vi "get trigger out before integration.vi"(8 "error in (no error)":errorcluster, 11 "LineCCD in":refnum<class "LineCCD.lvclass">) -> (0 "error out":errorcluster, 3 "LineCCD out":refnum<class "LineCCD.lvclass">)   [LabVIEW 2012, in "LineCCD.lvclass"]
uses:
  LineCCD.lvclass
  LineCCD.lvclass/LineCCD.ctl
  <instrlib>/ALPHALAS CCD S Series/ALPHALAS CCD S Series.lvlib
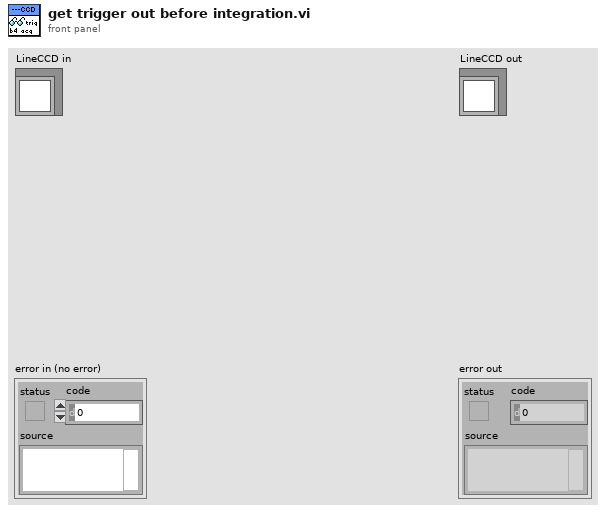
[diagram p1: front panel]
types:
  T1 = typedef "ALPHALAS CCD S Series.lvlib/Trig Out Before Integration.ctl" = u32
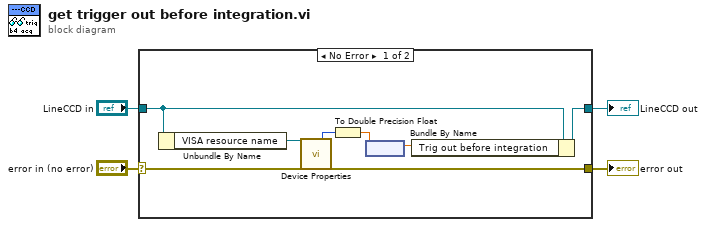
[diagram p0: block diagram]
diagram:
  n1 = case shown="No Error" "error in (no error)" {
    selector: "error in (no error)" -> [w7 w14]
    tunnel: [w6 w14] -> w3
    tunnel: [w8 w13] -> w1
    tunnel: "LineCCD in" -> [w9 w13]
    frame No Error {
      n2 = Unbundle By Name(w9) -> ("VISA resource name"=w10:refnum<visa-resource-name>)
      n3 = call <instrlib>:"Device Properties.vi"("VISA resource name"=w10, "error in (no error)"=w7) -> ("Trig Out Before Integration (µs)"=w5:T1, "error out"=w6:errorcluster)  [unwired: 6 in, 18 out]
      n4 = To Double Precision Float(number=w5) -> (double precision float=w11:dbl)
      n5 = node(w11) -> (w12:dbl[unit])
      n6 = Bundle By Name(cluster=w9, "Trig out before integration"=w12) -> (w8:refnum<class "LineCCD.lvclass">)
    }
    frame Error {
    }
  }
  "error out" <- w3
  "LineCCD out" <- w1
